vi "Get Unit Scaling.vi"(9 "Unit Index":u16, 10 "Quantity":T1=enum."Acceleration") -> (1 "Offset":dbl, 2 "Gain":dbl, 3 "Unit":string)   [LabVIEW 2011]
uses:
  Quantity enum.ctl
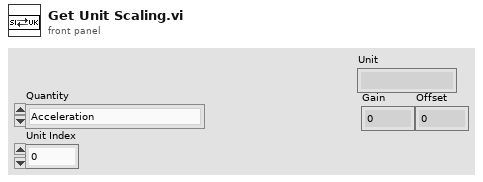
[diagram p1: front panel]
types:
  T1 = typedef "Quantity enum.ctl" = enum16{"NA", "Acceleration", "Angle", "Current", "Force", "Distance", "Pressure", "Resistance", "Rotational Speed", "Speed", "Temperature", "Tension", "Torque", "Voltage", "Weight"}
  T2 = cluster{"Available Units":cluster{"Unit":string, "Gain":dbl, "Offset":dbl}[]}[]
  T3 = cluster{"Available Units":cluster{"Unit":string, "Gain":dbl, "Offset":dbl}[]}
  T4 = cluster{"Unit":string, "Gain":dbl, "Offset":dbl}[]
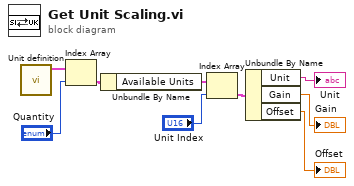
[diagram p0: block diagram]
diagram:
  n1 = call "Unit definition.vi"() -> ("Array"=w9:T2)  [unwired: 11 in]
  n2 = Index Array(array=w9, index="Quantity") -> (element=w8:T3)
  n3 = Unbundle By Name(w8) -> ("Available Units"=w6:T4)
  n4 = Index Array(array=w6, index="Unit Index") -> (element=w4:cluster{"Unit":string, "Gain":dbl, "Offset":dbl})
  n5 = Unbundle By Name(w4) -> ("Unit"=→"Unit":string, "Gain"=→"Gain":dbl, "Offset"=→"Offset":dbl)
